vi "parseHARO.vi"() -> ()   [LabVIEW 2013]
uses:
  <vilib>/regexp/Match Regular Expression.xnode
  <vilib>/Utility/file.llb/Write To Spreadsheet File (DBL).vi
panel:
  out "JSON string":string
  out "Parsed Haro":string[][](array[string])
  out "body out":string
  out "Array":string[](array[string])
  out "text":string
  in  "Raw email":path
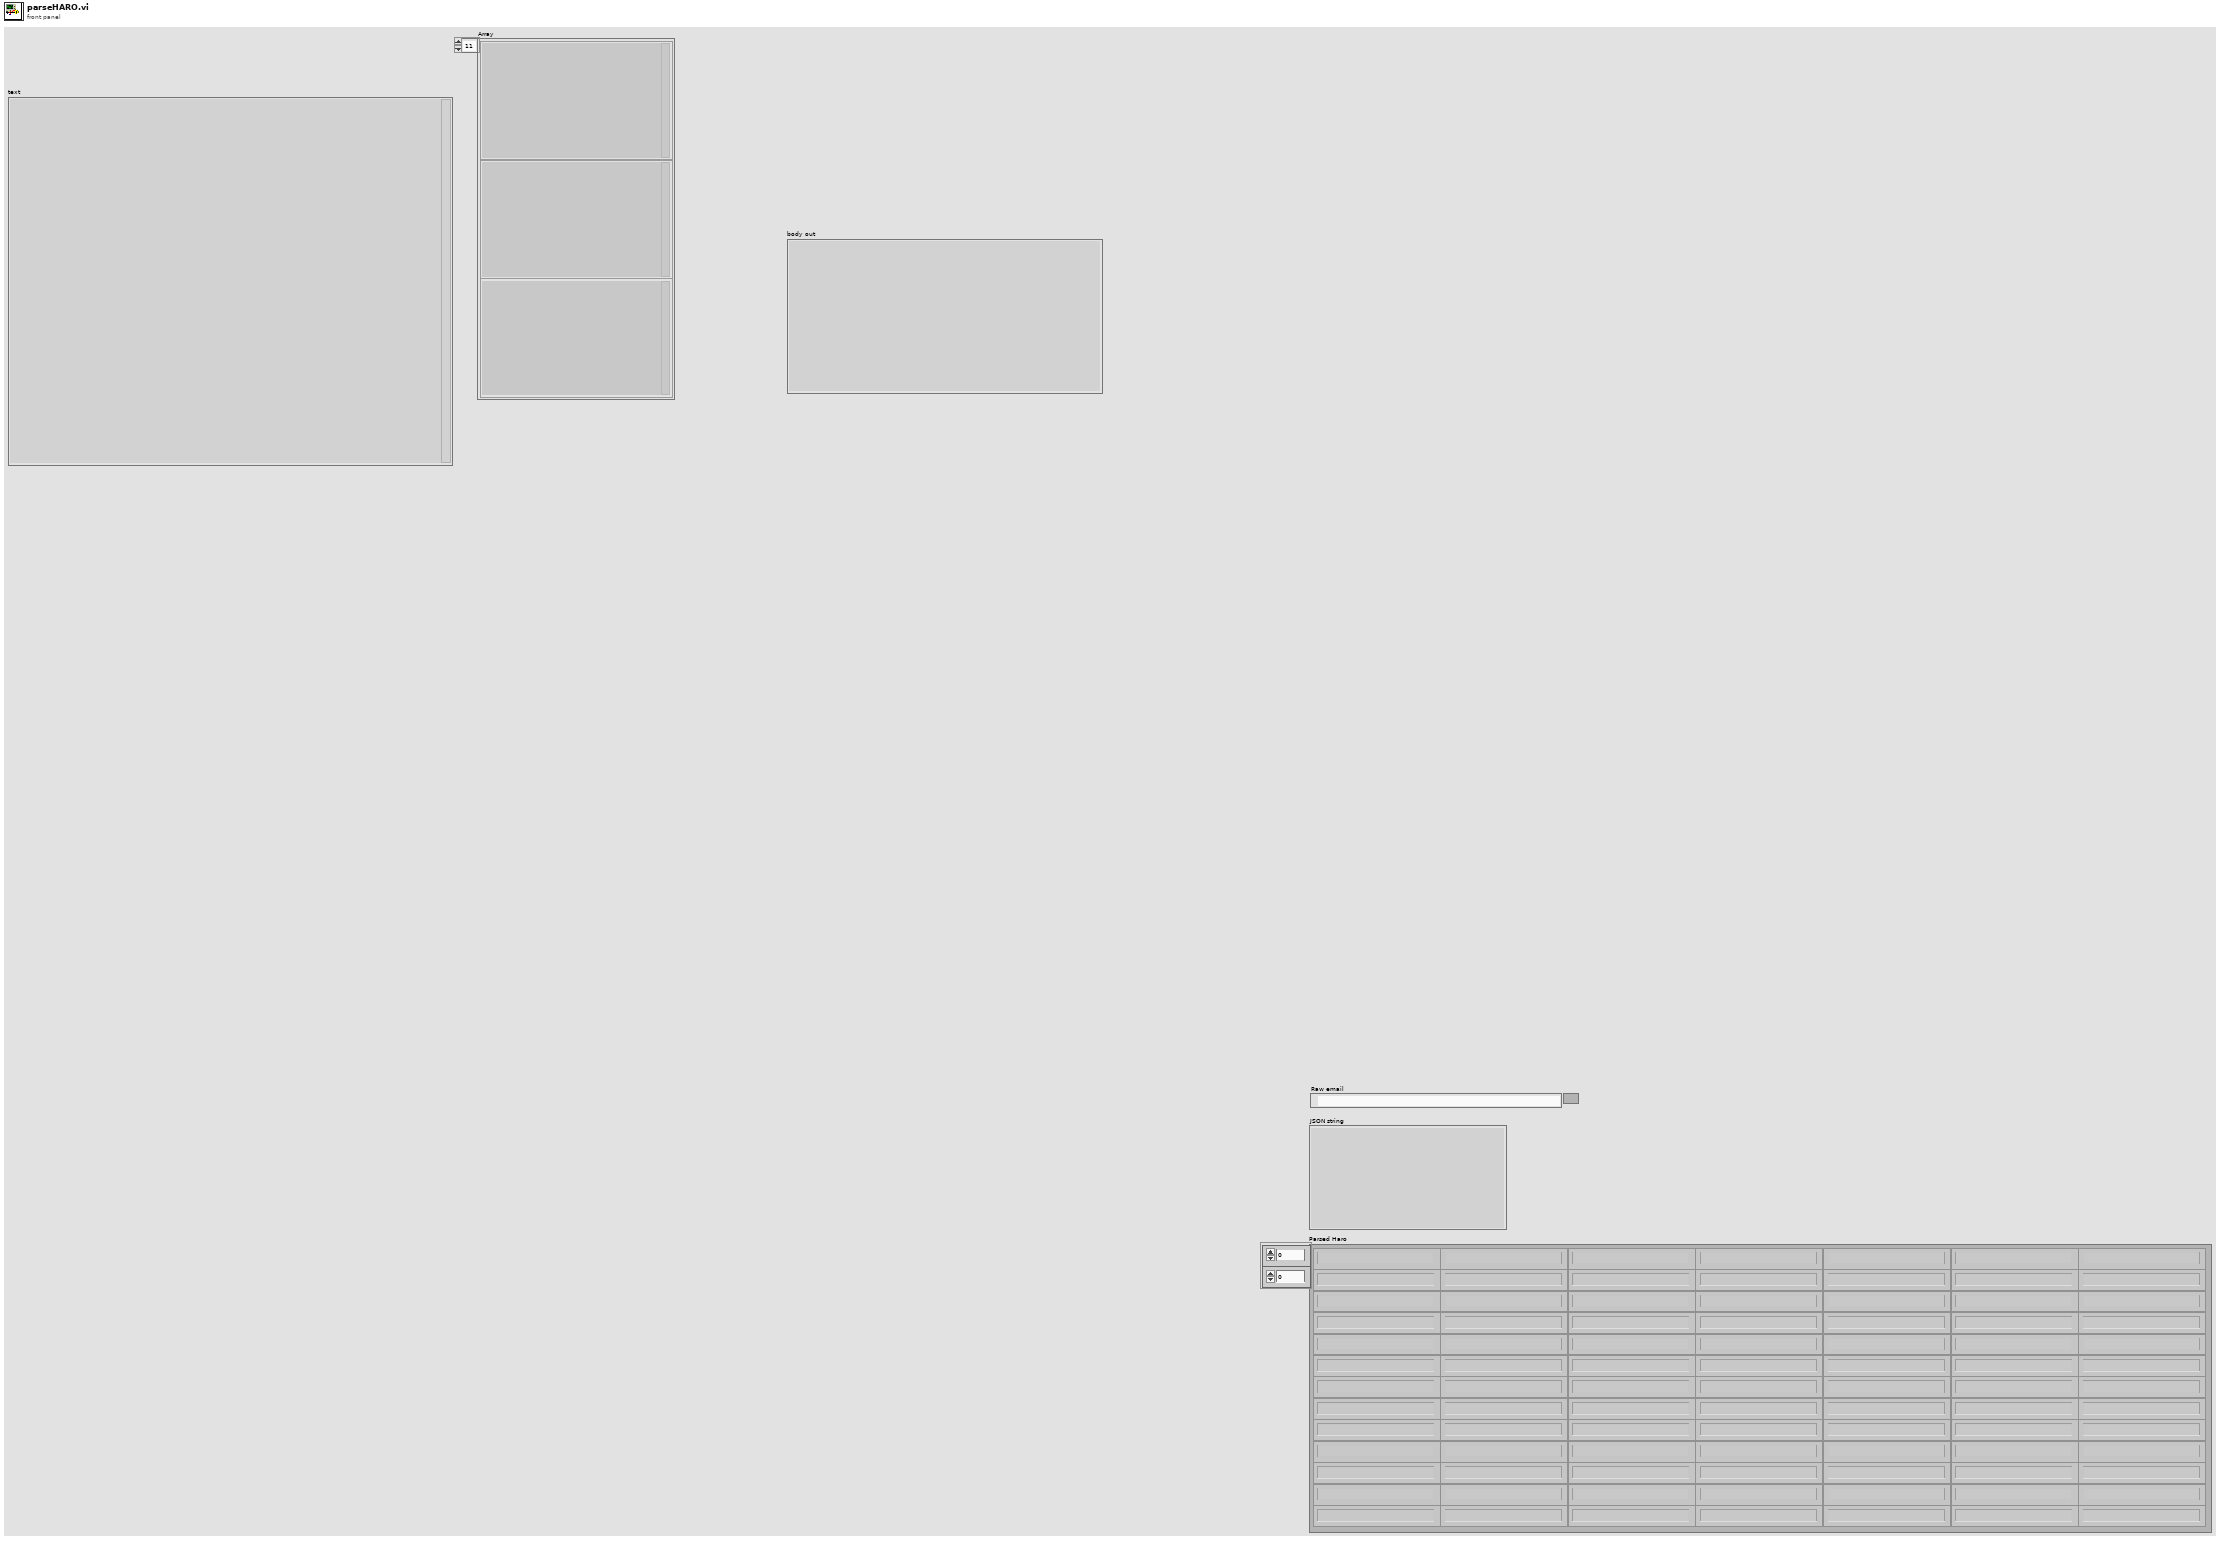
[diagram p1: front panel]
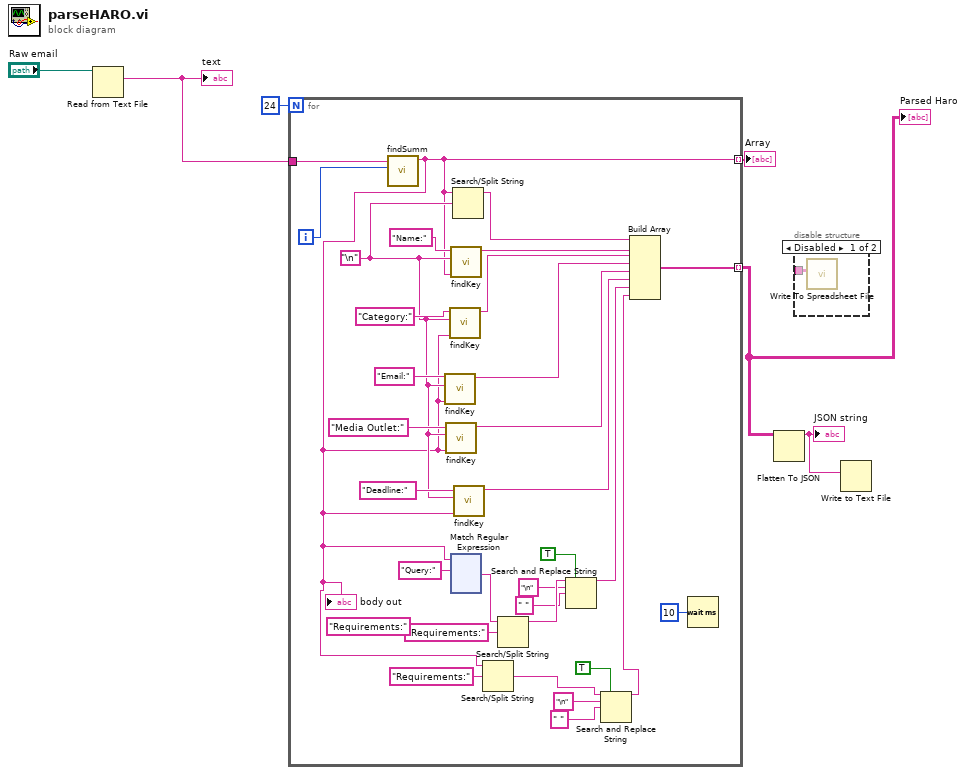
[diagram p0: block diagram]
diagram:
  n1 = Read from Text File(file (use dialog)="Raw email") -> (text=w5:string)  [unwired: 3 in, 3 out]
  "text" <- w5
  n2 = for {
    N: 24 -> [_]
    tunnel: [w17] -> w3 mode=indexing
    tunnel: w5 -> [w37]
    tunnel: [w22] -> w1 mode=indexing
    i -> [w36]
    (unwired) "Requirements:" ("Key")
    w29 = "\n"
    n3 = call "findSumm.vi"("#in"=w36, "body in in"=w37) -> ("body out"=w17:string)  [unwired: 9 in]
    "body out" <- w17
    n4 = call "findKey.vi"("Body In"=w17, "Cutoff Text"=w29, "Key"="Email:") -> ("Val out"=w25:string)  [unwired: 7 in, 1 out]
    n5 = call "findKey.vi"("Body In"=w17, "Cutoff Text"=w29, "Key"="Media Outlet:") -> ("Val out"=w24:string)  [unwired: 7 in, 1 out]
    n6 = call "findKey.vi"("Body In"=w17, "Cutoff Text"=w29, "Key"="Category:") -> ("Val out"=w26:string)  [unwired: 7 in, 1 out]
    n7 = call "findKey.vi"("Body In"=w17, "Cutoff Text"=w29, "Key"="Name:") -> ("Val out"=w27:string)  [unwired: 7 in, 1 out]
    n8 = xnode "Match Regular Expression"("input string"=w17, "regular expression"="Query:") -> ("after match"=w20:string)  [unwired: 4 in, 4 out]
    n9 = Search/Split String(string=w17, search string/char (-)=w29) -> (substring before match=w28:string)  [unwired: 1 in, 2 out]
    n10 = call "findKey.vi"("Body In"=w17, "Cutoff Text"=w29, "Key"="Deadline:") -> ("Val out"=w23:string)  [unwired: 7 in, 1 out]
    n11 = Search/Split String(string=w17, search string/char (-)="Requirements:") -> (match + rest of string=w8:string)  [unwired: 1 in, 2 out]
    n12 = Search/Split String(string=w20, search string/char (-)="Requirements:") -> (substring before match=w16:string)  [unwired: 1 in, 2 out]
    n13 = Search and Replace String(replace all?=TRUE ("replace all? (F)"), input string=w16, search string="\n", replace string=" " ("replace string (\"\")")) -> (result string=w13:string)  [unwired: 4 in, 3 out]
    n14 = Search and Replace String(replace all?=TRUE ("replace all? (F)"), input string=w8, search string="\n", replace string=" " ("replace string (\"\")")) -> (result string=w7:string)  [unwired: 4 in, 3 out]
    n15 = Build Array(w28, w27, w26, w25, w24, w23, w13, w7) -> (w22:string[])
    n16 = Wait (ms)(milliseconds to wait=u32 10) -> ()  [unwired: 1 out]
  }
  "Array" <- w3
  "Parsed Haro" <- w1
  n17 = Flatten To JSON(anything=w1) -> (JSON string=w2:string)  [unwired: 2 in, 1 out]
  "JSON string" <- w2
  n18 = disable-structure shown="Disabled" {
    disable-tunnel: _ -> [w152 _]
    frame Disabled {
      n19 = call-poly <vilib>:"Write To Spreadsheet File.vi"("2D data"=w152) -> ()  [unwired: 7 in, 1 out]
    }
    frame Enabled {
    }
  }
  n20 = Write to Text File(text=w2) -> ()  [unwired: 3 in, 3 out]
